vi "Write Pulse File.vi"(8 "error in (no error)":errorcluster, 9 "Open plot after pulse":bool, 10 "Pulse File":path, 11 "Monitor-Pulse in":refnum<class "Monitor-Pulse.lvclass">) -> (0 "error out":errorcluster, 3 "Monitor-Pulse out":refnum<class "Monitor-Pulse.lvclass">)   [LabVIEW 2016, in "Monitor-Pulse.lvclass"]
uses:
  Monitor-Pulse.lvclass
  Measure_core/Plots/Plot types.ctl
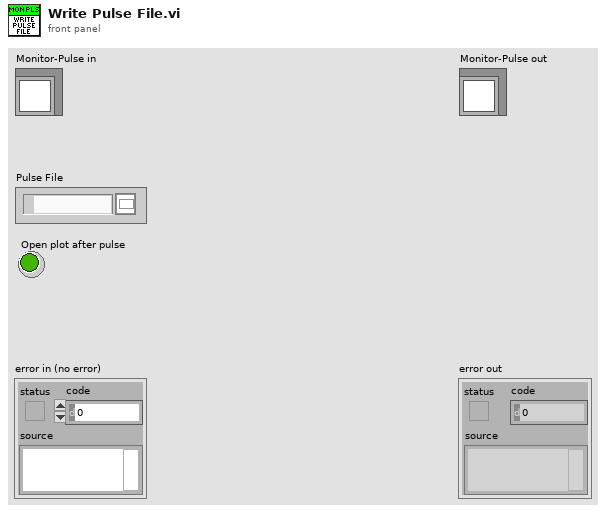
[diagram p1: front panel]
types:
  T1 = typedef "Plot types.ctl" = enum16{"Waveform Plot", "XY Plot", "Full XY"}
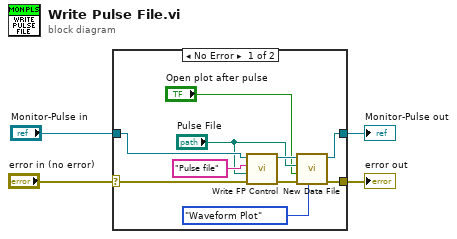
[diagram p0: block diagram]
diagram:
  n1 = case shown="No Error" "error in (no error)" {
    selector: "error in (no error)" -> [w12 w16]
    tunnel: [w8 w16] -> w3
    tunnel: [w10 w15] -> w1
    tunnel: "Monitor-Pulse in" -> [w14 w15]
    frame No Error {
      n2 = call-dynamic "Write FP Control.vi"("error in (no error)"=w12, "Control Value"="Pulse File", "Control Name"="Pulse file", "Measure Object in"=w14) -> ("error out"=w9:errorcluster, "Measure Object out"=w11:refnum<class "Monitor-Pulse.lvclass">)  [unwired: 6 in]
      n3 = call-dynamic "New Data File.vi"("Plot type"=Plot_types."Waveform Plot", "error in (no error)"=w9, "New plot if not open"="Open plot after pulse", "File"="Pulse File", "Application Controller in"=w11) -> ("error out"=w8:errorcluster, "Application Controller out"=w10:refnum<class "Monitor-Pulse.lvclass">)  [unwired: 5 in]
    }
    frame Error {
    }
  }
  "error out" <- w3
  "Monitor-Pulse out" <- w1
